vi "Stop Core.vi"(10 "final error code":i32, 11 "ErrorLog in":refnum<class "ErrorLog.lvclass">) -> (3 "ErrorLog out":refnum<class "ErrorLog.lvclass">)   [LabVIEW 2019, in "ErrorLog.lvlib" / "ErrorLog.lvclass"]
doc: "(<B>Filename</B>: Actor Framework.lvlib:Actor.lvclass:Stop Core.vi)\n\nDefines what the actor does before it stops. Use the <B>final error code</B> input to determine whether the actor shut down in response to an error.\n\nBy default, this method passes the Stop message along to all auto-stop nested actors. A descendant class may override this method to define additional behavior, such as shutting down any processes the actor initiated in its override of the Actor Core method."
uses:
  ErrorLog.lvclass
  LogsAbstract/LogsAbstract.lvclass
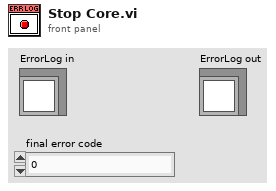
[diagram p1: front panel]
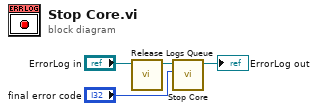
[diagram p0: block diagram]
diagram:
  n1 = call-dynamic "Release Logs Queue.vi"("EventLog in"="ErrorLog in") -> ("EventLog out"=w1:refnum<class "ErrorLog.lvclass">)  [unwired: 9 in, 1 out]
  n2 = call-parent "Stop Core.vi"("final error code"="final error code", "LogsAbstract in"=w1) -> ("LogsAbstract out"=→"ErrorLog out":refnum<class "ErrorLog.lvclass">)  [unwired: 9 in]
